vi "get save properties.vi"(8 "error in":errorcluster caption="错误输入（无错误）", 11 "PanelRootNode 输入":refnum<class "PanelRootNode.lvclass"> caption="DNL_LabVIEW Object in") -> (0 "error out":errorcluster caption="错误输出", 1 "Values":string[](array[string]), 2 "Names":string[](array[string]), 3 "PanelRootNode 输出":refnum<class "PanelRootNode.lvclass"> caption="DNL_LabVIEW Object out")   [LabVIEW 2016, in "PanelRootNode.lvclass"]
uses:
  PanelRootNode.lvclass
  C:/Users/CL/Desktop/ZcDAQprj0811/ZcDAQprj/Modules/DAQ-Display/PanelSplitToolkit/PanelDataNode/PanelDataNode.lvclass
  PanelDataNode/PanelDataNode.lvclass
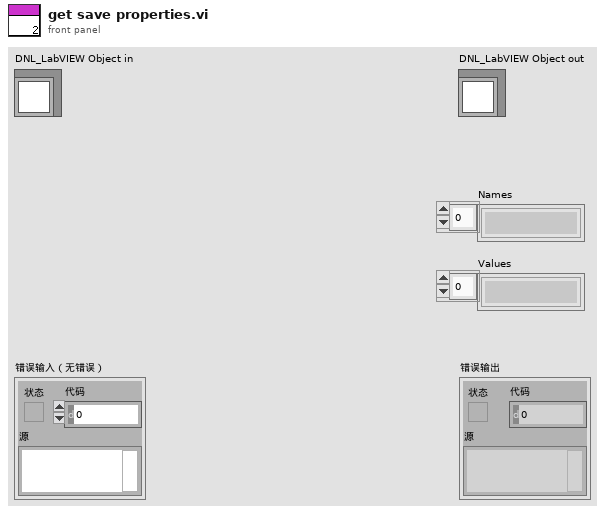
[diagram p1: front panel]
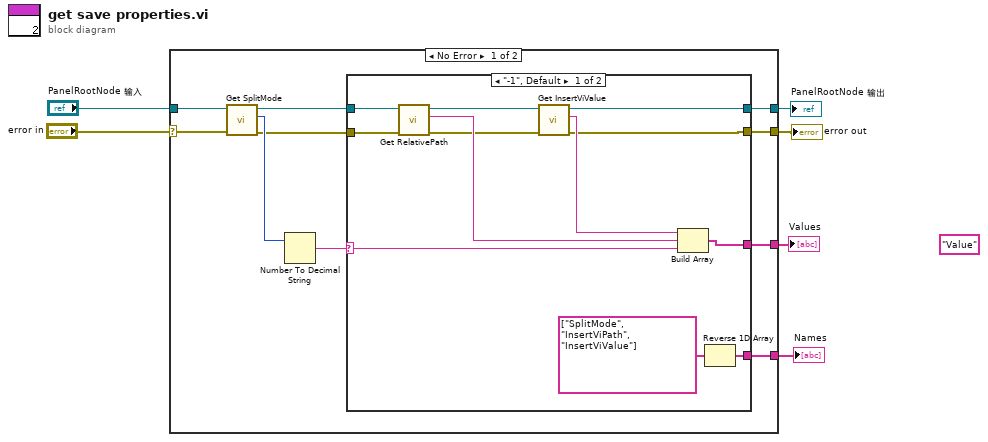
[diagram p0: block diagram]
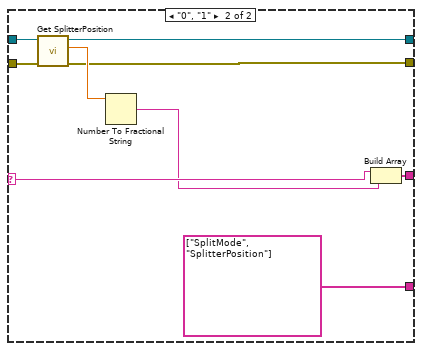
[diagram p2: hidden frame]
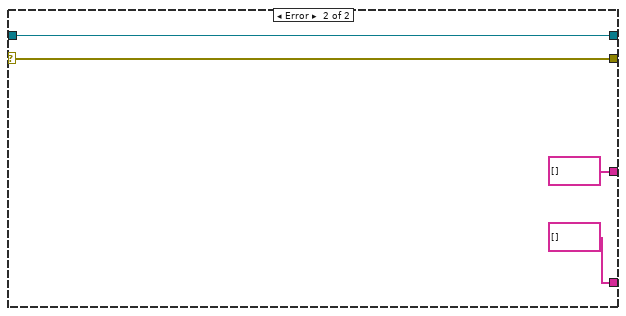
[diagram p3: hidden frame]
diagram:
  (unwired) "Value" ("元素")
  n1 = case shown="No Error" "error in" {
    selector: "error in" -> [w8 w41]
    tunnel: [w9 w41] -> w5
    tunnel: [w14 w40] -> w3
    tunnel: "PanelRootNode 输入" -> [w12 w40]
    tunnel: [w13 string[] []] -> w2
    tunnel: [w11 string[] []] -> w1
    frame No Error {
      n2 = call-dynamic "Get SplitMode.vi"("error in (no error)"=w8, "PanelDataNode 输入"=w12) -> ("error out"=w10:errorcluster, "Split Mode"=w16:i32, "PanelDataNode 输出"=w15:refnum<class "PanelRootNode.lvclass">)  [unwired: 7 in]
      n3 = Number To Decimal String(number=w16) -> (decimal integer string=w7:string)  [unwired: 1 in]
      n4 = case shown="\"-1\", Default" w7 {
        selector: w7 -> [w26 w31]
        tunnel: w15 -> [w28 w37]
        tunnel: [w19 w33] -> w14
        tunnel: [w25 w35] -> w13
        tunnel: [w22 string[] ["SplitMode", "SplitterPosition"]] -> w11
        tunnel: w10 -> [w27 w34]
        tunnel: [w17 w32] -> w9
        frame "-1", Default {
          n5 = call "Get RelativePath.vi"("error in (no error)"=w27, "PanelRootNode 输入"=w28) -> ("error out"=w18:errorcluster, "RelativePath"=w24:string, "PanelRootNode 输出"=w20:refnum<class "PanelRootNode.lvclass">)  [unwired: 7 in]
          n6 = call-dynamic "Get InsertViValue.vi"("error in (no error)"=w18, "PanelDataNode 输入"=w20) -> ("error out"=w17:errorcluster, "ViValue"=w21:string, "PanelDataNode 输出"=w19:refnum<class "PanelRootNode.lvclass">)  [unwired: 7 in]
          n7 = Build Array(w21, w24, w26) -> (w25:string[])
          n8 = Reverse 1D Array(array=string[] ["SplitMode", "InsertViPath", "InsertViValue"]) -> (reversed array=w22:string[])
        }
        frame "0", "1" {
          n9 = call "Get SplitterPosition.vi"("error in (no error)"=w34, "PanelDataNode 输入"=w37) -> ("error out"=w32:errorcluster, "SplitterPosition(relative)"=w36:dbl, "PanelDataNode 输出"=w33:refnum<class "PanelRootNode.lvclass">)  [unwired: 7 in]
          n10 = Number To Fractional String(number=w36) -> (F-format string=w30:string)  [unwired: 3 in]
          n11 = Build Array(w31, w30) -> (w35:string[])
        }
      }
    }
    frame Error {
    }
  }
  "error out" <- w5
  "PanelRootNode 输出" <- w3
  "Values" <- w2
  "Names" <- w1
